vi "DA output scale.vi"(8 "error in (no error)":errorcluster, 10 "j (0)":T1, 11 "VISA resource name":refnum<visa-resource-name>) -> (0 "error out":errorcluster, 3 "VISA resource name out":refnum<visa-resource-name>)   [LabVIEW 2015, in "SR400.lvlib"]
doc: "AM { j }\nIf j is included, the AM command sets the D/A\noutput scale. If j is absent, the D/A output scale is\nreturned.\nj Output scale\n0 Log (1V/decade)\n1 987######\n2 #876#####\n3 ##765####\n4 ###654###\n5 ####543##\n6 #####432#\n7 ######321"
uses:
  SR400.lvlib
  Typedefs/Output Scale.ctl
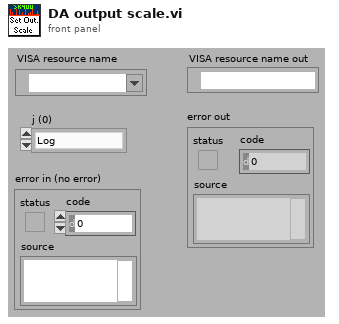
[diagram p1: front panel]
types:
  T1 = typedef "SR400.lvlib/Output Scale.ctl" = enum16{"Log", "987######", "#876#####", "##765####", "###654###", "####543##", "#####432#", "######321"}
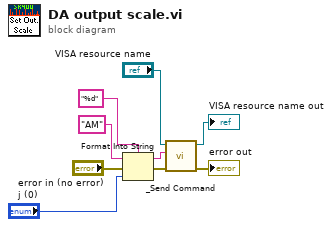
[diagram p0: block diagram]
diagram:
  n1 = Format Into String(format string="%d", initial string="AM" ("command"), error in="error in (no error)", "j (0)") -> (resulting string=w5:string, error out=w4:errorcluster)
  n2 = call "_Send Command.vi"("error in (no error)"=w4, "Command"=w5, "VISA resource name"="VISA resource name") -> ("error out"=→"error out":errorcluster, "VISA resource name out"=→"VISA resource name out":refnum<visa-resource-name>)  [unwired: 1 in, 6 out]
